vi "LongpressButton.vi"(1 "Threshold (ms)":u32=100, 2 "Button":bool) -> (0 "Longpress Button":bool)   [LabVIEW 2019]
doc: "This VI takes as input a Boolean button press, and only returns TRUE if the button has been held continuously for longer than the specified time threshold."
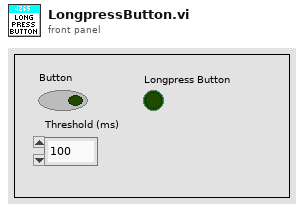
[diagram p1: front panel]
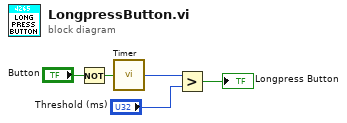
[diagram p0: block diagram]
diagram:
  n1 = Not(x="Button") -> (.not. x?=w4:bool)
  n2 = call "Timer.vi"("Reset Timer"=w4) -> ("Time (ms)"=w3:u32)
  n3 = Greater?(x=w3, y="Threshold (ms)") -> (0:→"Longpress Button":bool)
